vi "WPI_RobotDriveRotateVector.vi"(8 "Angle":dbl, 10 "X":dbl, 11 "Y":dbl) -> (2 "X'":dbl, 3 "Y'":dbl)   [LabVIEW 2017]
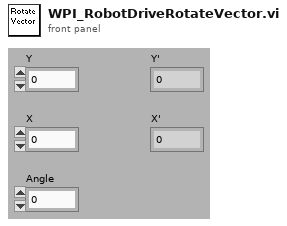
[diagram p1: front panel]
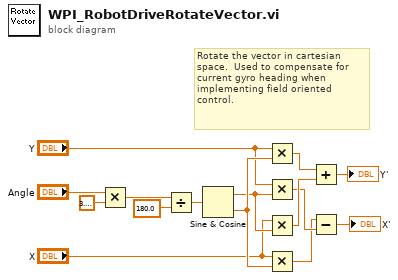
[diagram p0: block diagram]
diagram:
  # "Rotate the vector in cartesian space.  Used to compensate for current gyro heading when implementing field oriented control."
  n1 = Multiply(x="Angle", y=3.141592653589793) -> (x*y=w3:dbl)
  n2 = Divide(x=w3, y=180.0) -> (x/y=w5:dbl)
  n3 = Sine & Cosine(0:w5) -> (1:w10:dbl, 2:w12:dbl)
  n4 = Multiply(x="Y", y=w12) -> (x*y=w13:dbl)
  n5 = Multiply(x="Y", y=w10) -> (x*y=w7:dbl)
  n6 = Multiply(x="X", y=w10) -> (x*y=w14:dbl)
  n7 = Multiply(x="X", y=w12) -> (x*y=w6:dbl)
  n8 = Add(x=w13, y=w14) -> (x+y=→"Y'":dbl)
  n9 = Subtract(x=w6, y=w7) -> (x-y=→"X'":dbl)
